vi "SQLite Add Transaction Test.vi"(8 "Error In (no error)":errorcluster, 11 "DB Operator In":refnum<class "DB Operator.lvclass">) -> (0 "Error Out":errorcluster, 3 "DB Operator Out":refnum<class "DB Operator.lvclass">)   [LabVIEW 2023]
uses:
  DB Operator/DB Operator.lvclass
  SQLite DB Operator/SQLite DB Operator.lvclass
  H:/Desktop/LabVIEW/LabView Repo/Expense Tracker DB Operator/DB Operator/DB Operator.lvclass
  DB Operator/Public/Ctrls/DB Controls/Transaction.ctl
  SQLite DB Operator/SQLite DB Operator.lvclass/SQLite DB Operator.ctl
  <vilib>/drjdpowell/SQLite Library/SQL Connection/Execute SQL (Variant Cluster results).vi
  <vilib>/addons/_JKI Toolkits/Caraya/classes/Assert/Assert Equal Value_Variant.vi
  <vilib>/addons/_JKI Toolkits/Caraya/classes/Assert/Assert Not Equal Value_Variant.vi
  <vilib>/drjdpowell/SQLite Library/SQL Connection/Connection.lvclass
  <vilib>/addons/_JKI Toolkits/Caraya/classes/Test/Test.lvclass
  <vilib>/drjdpowell/SQLite Library/SQLite.lvlib
  <vilib>/addons/_JKI Toolkits/Caraya/classes/Assert/Assert.lvclass
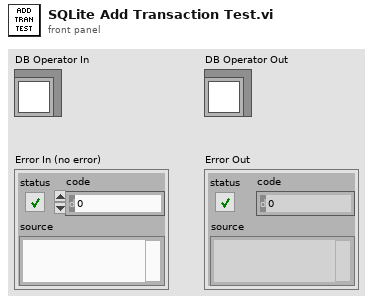
[diagram p1: front panel]
types:
  T1 = typedef "DB Operator.lvclass/Transaction.ctl" = cluster{"ID":u32, "Name":string, "Is Income":bool, "Value":dbl, "Amount":dbl, "Total":dbl, "Date of Entry":timestamp, "Date":timestamp, "Last Update":timestamp, "Category":u32, "Subcategory":u32, "Cycle":u32, "Description":string}
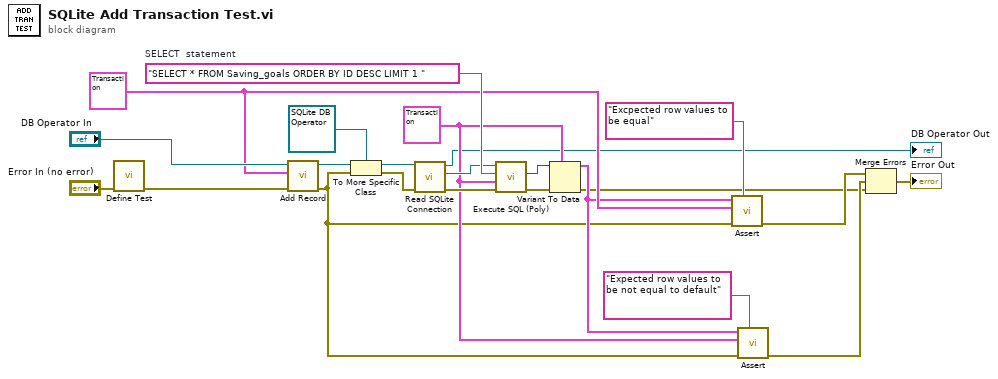
[diagram p0: block diagram]
diagram:
  w9 = T1 {"ID"=0, "Name"="", "Is Income"=FALSE, "Value"=0.0, "Amount"=0.0, "Total"=0.0, "Date of Entry"=timestamp(0 s since 1904-01-01), "Date"=timestamp(0 s since 1904-01-01), "Last Update"=timestamp(0 s since 1904-01-01), "Category"=0, "Subcategory"=0, "Cycle"=0, "Description"=""} ("Transaction")
  w8 = T1 {"ID"=1, "Name"="TestTran", "Is Income"=FALSE, "Value"=10.0, "Amount"=2.0, "Total"=20.0, "Date of Entry"=timestamp(3789590400 s since 1904-01-01), "Date"=timestamp(3786912000 s since 1904-01-01), "Last Update"=timestamp(3786912000 s since 1904-01-01), "Category"=1, "Subcategory"=1, "Cycle"=1, "Description"="TestDesc"} ("Transaction")
  w18 = "SELECT * FROM Saving_goals ORDER BY ID DESC LIMIT 1 "  # SELECT  statement
  n1 = call <vilib>:"Define Test.vi"("error in (no error)"="Error In (no error)") -> ("error out"=w19:errorcluster)  [unwired: 9 in, 1 out]
  n2 = call-dynamic "Add Record.vi"("Error In (no error)"=w19, "Data"=w8, "DB Operator in"="DB Operator In") -> ("Error Out"=w5:errorcluster, "DB Operator out"=w22:refnum<class "DB Operator.lvclass">)  [unwired: 7 in]
  n3 = To More Specific Class(target class=refnum<class "SQLite DB Operator.lvclass"> refnum ("SQLite DB Operator.lvclass"), reference=w22, error in=w5) -> (specific class reference=w21:refnum<class "SQLite DB Operator.lvclass">, error out=w10:errorcluster)
  n4 = call "Read SQLite Connection.vi"("Error In (no error)"=w10, "SQLite DB Operator In"=w21) -> ("Error Out"=w16:errorcluster, "SQLite.lvlib:Connection"=w17:refnum<class "Connection.lvclass">, "SQLite DB Operator out"=→"DB Operator Out":refnum<class "SQLite DB Operator.lvclass">)  [unwired: 7 in]
  n5 = call-poly <vilib>:"Execute SQL (Poly).vi"("error in (no error)"=w16, "Cluster"=w9, "SQL"=w18, "SQLite Connection in"=w17) -> ("error out"=w14:errorcluster, "Result (use Variant to Data)"=w13:variant)  [unwired: 5 in, 1 out]
  n6 = Variant To Data(error in=w14, type=w9, Variant=w13) -> (data=w6:T1, error out=w2:errorcluster)
  n7 = call-poly <vilib>:"Assert.vi"("Label"="Excpected row values to be equal" ("Label (VI Title)"), "error in (no error)"=w5, "Y"=w8, "X"=w6) -> ("error out"=w11:errorcluster)  [unwired: 6 in, 1 out]
  n8 = call-poly <vilib>:"Assert.vi"("Label"="Expected row values to be not equal to default" ("Label (VI Title)"), "error in (no error)"=w5, "Y"=w9, "X"=w6) -> ("error out"=w3:errorcluster)  [unwired: 6 in, 1 out]
  n9 = Merge Errors(w11, w3, w2) -> (→"Error Out":errorcluster)
